vi "Count Steps from Accel_SubVI.vi"(9 "width":i32, 10 "threshold":dbl, 11 "Queue Elements In":T1[](array[typedef])) -> (1 "Pulse Array":dbl[](array[numeric]), 2 "Step Count":i32, 3 "Step Indices":i32[](array[numeric]))   [LabVIEW 2021]
uses:
  ProducerConsumer Data Cluster_TDef.ctl
  <vilib>/Analysis/NI_AALPro.lvlib
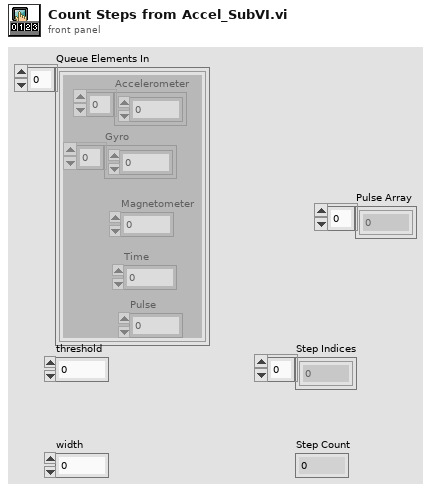
[diagram p1: front panel]
types:
  T1 = typedef "ProducerConsumer Data Cluster_TDef.ctl" = cluster{"Accelerometer":dbl[], "Gyro":dbl[], "Magnetometer":dbl, "Time":i32, "Pulse":dbl}
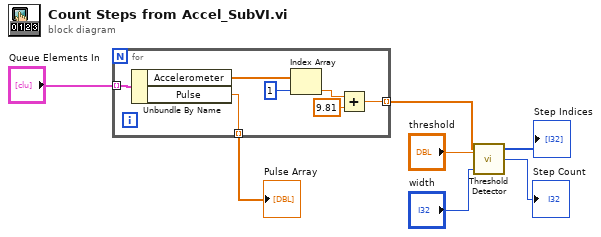
[diagram p0: block diagram]
diagram:
  n1 = for {
    tunnel: [w13] -> w4 mode=indexing
    tunnel: "Queue Elements In" -> [w11] mode=indexing
    tunnel: [w8] -> w1 mode=indexing
    n2 = Unbundle By Name(w11) -> ("Accelerometer"=w10:dbl[], "Pulse"=w8:dbl)
    n3 = Index Array(array=w10, index=1) -> (element=w9:dbl)
    n4 = Add(x=w9, y=9.81 ("x")) -> (x+y=w13:dbl)
  }
  "Pulse Array" <- w1
  n5 = call <vilib>:"Threshold Detector.vi"("width"="width", "threshold"="threshold", "X"=w4) -> ("count"=→"Step Count":i32, "Indices"=→"Step Indices":i32[])  [unwired: 1 out]
